vi "MG369X_init.vi"(2 "error in (no error)":errorcluster, 3 "MG369X_control":T1={"Initial Frequency (Hz)"=2000000000.0, "Initial Power Level (dBm)"=20.0, "Trigger Type (1: Free Run)"=1, "Clock Rate (4: Clock 100)"=4, "Trigger Edge Type (0: Trigger Rising)"=0, "Polarity (1: High RF On)"=1, "Pulse_Period (s)"=1e-08, "Mode (1: Single)"=1, "Reset (True)"=TRUE, "ID Query (True)"=TRUE} {"Mode (1: Single)" items=["Single"=1, "Doublet"=2, "Triplet"=3, "Quadruplet"=4]; "Pulse_Period (s)" format="%#_12g"; "Polarity (1: High RF On)" items=["Low RF On", "High RF On"]; "Trigger Edge Type (0: Trigger Rising)" items=["Trigger Rising", "Trigger Falling"]; "Clock Rate (4: Clock 100)" items=["Clock 10"=1, "Clock 100"=4]; "Trigger Type (1: Free Run)" items=["Free Run"=1, "Gated"=2, "Delayed"=3, "Triggered"=4, "Triggered w/delay"=5]}, 4 "MG369X_VISA":refnum<visa-resource-name>="GPIB0::5::INSTR") -> (0 "error out":errorcluster, 1 "MG369X_Visa_out":refnum<visa-resource-name>)   [LabVIEW 2020]
uses:
  <instrlib>/Anritsu MG369X Series/Anritsu MG369X Series.lvlib
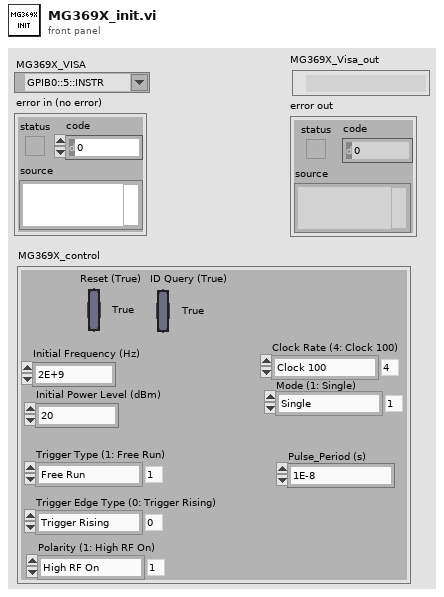
[diagram p1: front panel]
types:
  T1 = cluster{"Initial Frequency (Hz)":dbl, "Initial Power Level (dBm)":dbl, "Trigger Type (1: Free Run)":u16, "Clock Rate (4: Clock 100)":u16, "Trigger Edge Type (0: Trigger Rising)":u16, "Polarity (1: High RF On)":u16, "Pulse_Period (s)":dbl, "Mode (1: Single)":u16, "Reset (True)":bool, "ID Query (True)":bool}
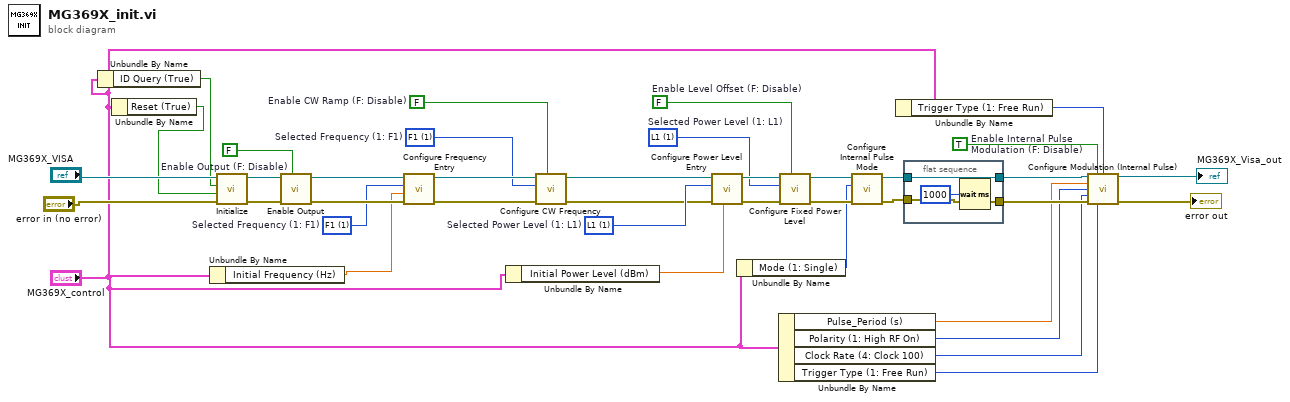
[diagram p0: block diagram]
diagram:
  w23 = TRUE  # Enable Internal Pulse Modulation (F: Disable)
  w22 = FALSE  # Enable CW Ramp (F: Disable)
  w25 = u16 1 items=["F0", "F1", "F2", "F3", "F4", "F5", "F6", "F7", "F8", "F9", "M0", "M1", "M2", "M3", "M4", "M5", "M6", "M7", "M8", "M9"]  # Selected Frequency (1: F1)
  w24 = FALSE  # Enable Level Offset (F: Disable)
  w30 = u16 1 items=["L0", "L1", "L2", "L3", "L4", "L5", "L6", "L7", "L8", "L9"]  # Selected Power Level (1: L1)
  w33 = u16 1 items=["L0", "L1", "L2", "L3", "L4", "L5", "L6", "L7", "L8", "L9"]  # Selected Power Level (1: L1)
  w34 = u16 1 items=["F0", "F1", "F2", "F3", "F4", "F5", "F6", "F7", "F8", "F9", "M0", "M1", "M2", "M3", "M4", "M5", "M6", "M7", "M8", "M9"]  # Selected Frequency (1: F1)
  w37 = FALSE  # Enable Output (F: Disable)
  n1 = Unbundle By Name("MG369X_control") -> ("ID Query (True)"=w3:bool)
  n2 = Unbundle By Name("MG369X_control") -> ("Reset (True)"=w1:bool)
  n3 = Unbundle By Name("MG369X_control") -> ("Initial Frequency (Hz)"=w11:dbl)
  n4 = call <instrlib>:"Initialize.vi"("error in (no error)"="error in (no error)", "Reset (True)"=w1, "ID Query (True)"=w3, "VISA resource name"="MG369X_VISA") -> ("error out"=w39:errorcluster, "VISA resource name out"=w38:refnum<visa-resource-name>)  [unwired: 6 in]
  n5 = call <instrlib>:"Enable Output.vi"("Enable Output (F: Disable)"=w37, "error in (no error)"=w39, "VISA resource name"=w38) -> ("error out"=w35:errorcluster, "VISA resource name out"=w36:refnum<visa-resource-name>)  [unwired: 7 in]
  n6 = call <instrlib>:"Configure Frequency Entry.vi"("error in (no error)"=w35, "Frequency (2.2E+9 Hz)"=w11, "Selected Frequency (1: F1)"=w34, "VISA resource name"=w36) -> ("error out"=w28:errorcluster, "VISA resource name out"=w29:refnum<visa-resource-name>)  [unwired: 6 in]
  n7 = Unbundle By Name("MG369X_control") -> ("Initial Power Level (dBm)"=w10:dbl)
  n8 = call <instrlib>:"Configure CW Frequency.vi"("Enable CW Ramp (F: Disable)"=w22, "error in (no error)"=w28, "Selected Frequency (1: F1)"=w25, "VISA resource name"=w29) -> ("error out"=w26:errorcluster, "VISA resource name out"=w27:refnum<visa-resource-name>)  [unwired: 6 in]
  n9 = call <instrlib>:"Configure Power Level Entry.vi"("Power Level (0.0 DM or VT or SPS)"=w10, "error in (no error)"=w26, "Selected Power Level (1: L1)"=w33, "VISA resource name"=w27) -> ("error out"=w31:errorcluster, "VISA resource name out"=w32:refnum<visa-resource-name>)  [unwired: 6 in]
  n10 = Unbundle By Name("MG369X_control") -> ("Mode (1: Single)"=w5:u16)
  n11 = Unbundle By Name("MG369X_control") -> ("Pulse_Period (s)"=w6:dbl, "Polarity (1: High RF On)"=w7:u16, "Clock Rate (4: Clock 100)"=w8:u16, "Trigger Type (1: Free Run)"=w9:u16)
  n12 = call <instrlib>:"Configure Fixed Power Level.vi"("Enable Level Offset (F: Disable)"=w24, "error in (no error)"=w31, "Selected Power Level (1: L1)"=w30, "VISA resource name"=w32) -> ("error out"=w20:errorcluster, "VISA resource name out"=w21:refnum<visa-resource-name>)  [unwired: 6 in]
  n13 = call <instrlib>:"Configure Internal Pulse Mode.vi"("error in (no error)"=w20, "Mode (1: Single)"=w5, "VISA resource name"=w21) -> ("error out"=w16:errorcluster, "VISA resource name out"=w18:refnum<visa-resource-name>)  [unwired: 7 in]
  n14 = Unbundle By Name("MG369X_control") -> ("Trigger Type (1: Free Run)"=w4:u16)
  n15 = flat-sequence {
    tunnel: [w42] -> w19
    tunnel: w18 -> [w42]
    tunnel: [w41] -> w17
    tunnel: w16 -> [w41]
    frame #0 {
      n16 = Wait (ms)(milliseconds to wait=u32 1000) -> ()  [unwired: 1 out]
    }
  }
  n17 = call <instrlib>:"Configure Modulation (Internal Pulse).vi"("VISA resource name"=w19, "Enable Internal Pulse Modulation (F: Disable)"=w23, "Trigger Edge Type (0: Trigger Rising)"=w4, "Period (1.0E-8 Second)"=w6, "Polarity (1: High RF On)"=w7, "Clock Rate (4: Clock 100)"=w8, "error in (no error)"=w17, "Trigger Type (1: Free Run)"=w9) -> ("VISA resource name out"=→"MG369X_Visa_out":refnum<visa-resource-name>, "error out"=→"error out":errorcluster)  [unwired: 6 in]
